vi "PlotPathSup.vi"(10 "Display":T5={"Mode"=enum."Inherit Value", "PointSize"=1.0, "LineWidth"=1.0}, 11 "PathSups":T1[](array[typedef])) -> ()   [LabVIEW 2014]
uses:
  TypeDefs/PathSupreme.ctl
  PSup2SCAN/Sub/VelocityProfile.ctl
  PSup2SCAN/Sub/PathCut.ctl
  PSup2SCAN/Sub/Segment.ctl
  ColorMaps.ctl
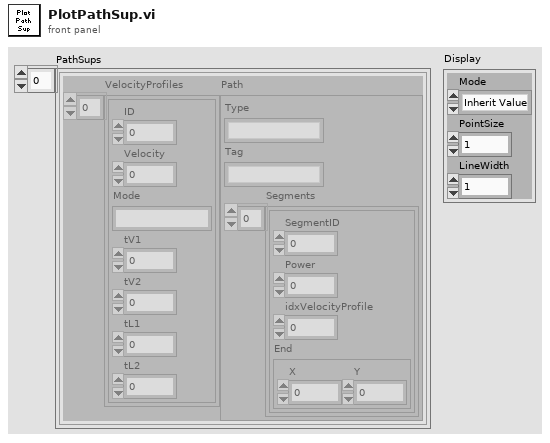
[diagram p1: front panel]
types:
  T1 = typedef "PathSupreme.ctl" = cluster{"VelocityProfiles":T2[], "Path":T3}
  T2 = typedef "VelocityProfile.ctl" = cluster{"ID":u32, "Velocity":dbl, "Mode":string, "tV1":u32, "tV2":u32, "tL1":u32, "tL2":u32}
  T3 = typedef "PathCut.ctl" = cluster{"Type":string, "Tag":string, "Segments":T4[]}
  T4 = typedef "Segment.ctl" = cluster{"SegmentID":u16, "Power":sgl, "idxVelocityProfile":u16, "End":cluster{"X":sgl, "Y":sgl}}
  T5 = cluster{"Mode":enum16{"Inherit Value", "Points", "Wireframe", "Polygons"}, "PointSize":sgl, "LineWidth":sgl}
  T6 = typedef "ColorMaps.ctl" = u16
  T7 = typedef "Point3D.ctl" = cluster{"X":sgl, "Y":sgl, "Z":sgl}
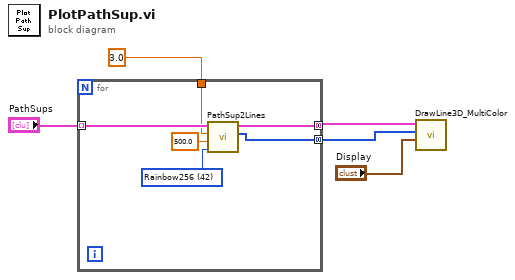
[diagram p0: block diagram]
diagram:
  n1 = for {
    tunnel: [w9] -> w3 mode=concatenating
    tunnel: [w8] -> w2 mode=concatenating
    tunnel: "PathSups" -> [w7] mode=indexing
    tunnel: 3.0 ("Z") -> [w6]
    w10 = T6 42 items=["Bathymetry9", "BlackBody", "Blue", "BlueBlackRed", "BlueGreenOrange", "BlueHot", "BlueHot256", "BlueRedGreen", "BlueRedGreen256", "BrownViolet", "Classification", "ColdWarm", "Copper", "Cyan", "CyanMagenta", "Cycles", "dBZ14", "dBZ21", "EOSOrangeBlue11", "EOSSpectral11", "Fiddle", "Geo", "Geo32", "Gold", "Grays", "Grays16", "Grays256", "Green", "GreenMagenta16", "LandAndSea", "LandAndSea8", "Magenta", "Mocha", "Mud", "Pastels", "PastelsMap", "PastelsMap20", "PlanetEarth", "PlanetEarth256", "Rainbow", "Rainbow4Cycles", "Rainbow16", "Rainbow256", "RainbowCycle", "Red", "RedWhiteBlue", "RedWhiteBlue256", "RedWhiteGreen", "Relief", "Relief19", "SeaLandAndFire", "Spectrum", "SpectrumBlack", "Terrain", "Terrain256", "VioletOrangeYellow", "Web216", "Yellow", "YellowHot", "YellowHot256"] ("ColorMap")
    n2 = call "PathSup2Lines.vi"("ColorMap"=w10, "HighPower"=500.0, "Z"=w6, "PathSupreme"=w7) -> ("Colors"=w8:u32[], "Lines"=w9:cluster{"P0":T7, "P1":T7}[])  [unwired: 6 in]
  }
  n3 = call "DrawLine3D_MultiColor.vi"("Display"="Display", "Colors"=w2, "Lines"=w3) -> ()  [unwired: 9 in]
